vi "Solution part 2.vi"() -> ()   [LabVIEW 2020]
panel:
  out "pt 1 solution":u64
  out "first index":i32
  out "last index":i32
  out "result":u64
  in  "data?":bool
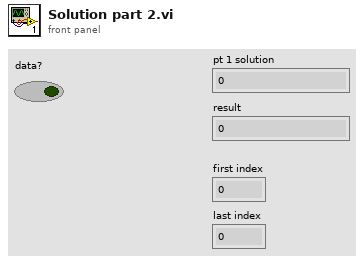
[diagram p1: front panel]
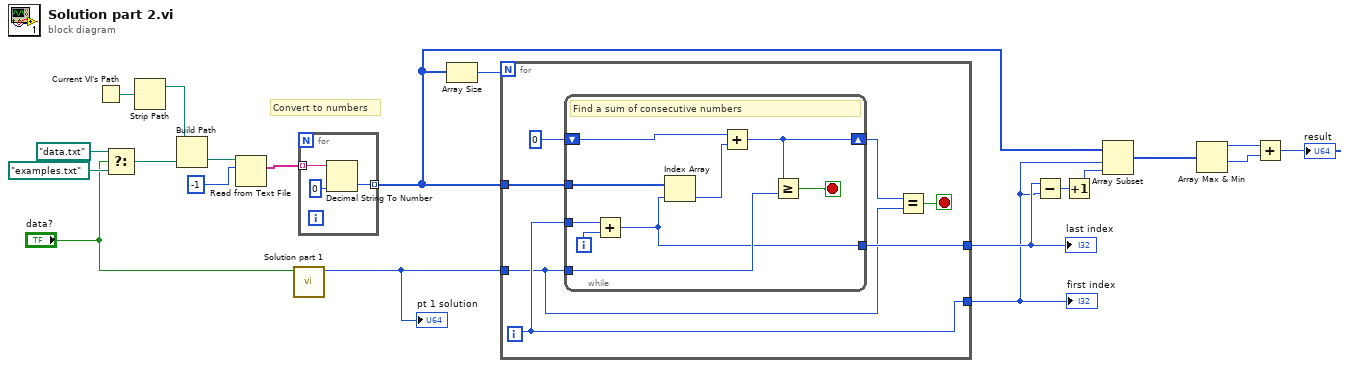
[diagram p0: block diagram]
diagram:
  # "Convert to numbers"
  n1 = Current VI's Path() -> (path=w17:path)
  n2 = Select(t=path "data.txt", s="data?", f=path "examples.txt") -> (s? t:f=w18:path)
  n3 = Strip Path(path=w17) -> (stripped path=w16:path)  [unwired: 1 out]
  n4 = Build Path(base path=w16, name or relative path=w18) -> (appended path=w15:path)
  n5 = Read from Text File(file (use dialog)=w15, count=-1) -> (text=w13:string[])  [unwired: 2 in, 3 out]
  n6 = call "Solution part 1.vi"("data?"="data?") -> ("result"=w11:u64)  [unwired: 10 in]
  "pt 1 solution" <- w11
  n7 = for {
    tunnel: w13 -> [w23] mode=indexing
    tunnel: [w21] -> w8 mode=indexing
    n8 = Decimal String To Number(string=w23, default (0L)=u64 0 ("count")) -> (number=w21:u64)  [unwired: 1 in, 1 out]
  }
  n9 = Array Size(array=w8) -> (size(s)=w10:i32)
  n10 = for {
    N: w10 -> [_]
    tunnel: w11 -> [w26]
    tunnel: w8 -> [w30]
    tunnel: [w28] -> w6
    tunnel: [w27] -> w7
    i -> [w28]
    stop <- w24 stop-if-true
    n11 = while {
      tunnel: w26 -> [w35]
      tunnel: w30 -> [w39]
      tunnel: w28 -> [w38]
      shift-right: [w34] -> w25
      shift-left: u64 0 ("count") -> [w37]
      tunnel: [w31] -> w27
      i -> [w33]
      stop <- w32 stop-if-true
      # "Find a sum of consecutive numbers"
      n12 = Add(x=w38, y=w33) -> (x+y=w31:i32)
      n13 = Index Array "Index Array"(array=w39, index=w31) -> (element=w36:u64)
      n14 = Add(x=w37, y=w36) -> (x+y=w34:u64)
      n15 = Greater Or Equal?(x=w34, y=w35) -> (x >= y?=w32:bool)
    }
    n16 = Equal?(x=w25, y=w26) -> (x = y?=w24:bool)
  }
  "last index" <- w7
  "first index" <- w6
  n17 = Subtract(x=w7, y=w6) -> (x-y=w4:i32)
  n18 = Increment(x=w4) -> (x+1=w5:i32)
  n19 = Array Subset "Array Subset"(array=w8, index=w6, length=w5) -> (w3:u64[])
  n20 = Array Max & Min(array=w3) -> (max value=w2:u64, min value=w1:u64)  [unwired: 2 out]
  n21 = Add(x=w2, y=w1) -> (x+y=→"result":u64)
